vi "Read Body.vi"(8 "error in (no error)":errorcluster, 11 "Request in":refnum<class "Request.lvclass">) -> (0 "error out":errorcluster, 3 "Request out":refnum<class "Request.lvclass">)   [LabVIEW 2023, in "Request.lvclass"]
uses:
  Request.lvclass
  Request.lvclass/Request.ctl
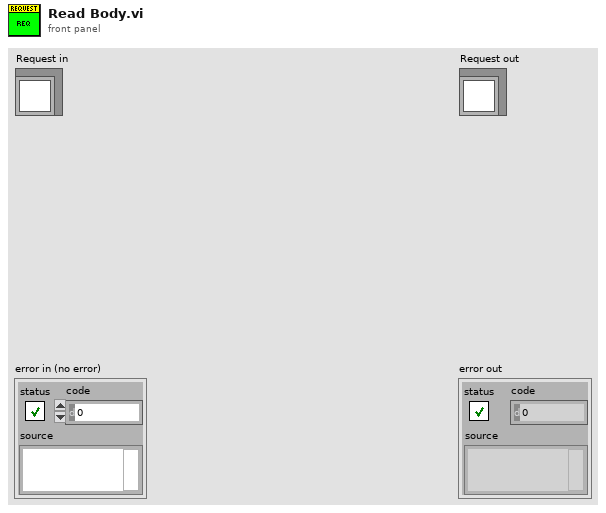
[diagram p1: front panel]
types:
  T1 = enum16{"Standard", "Buffered", "CRLF", "Immediate"}
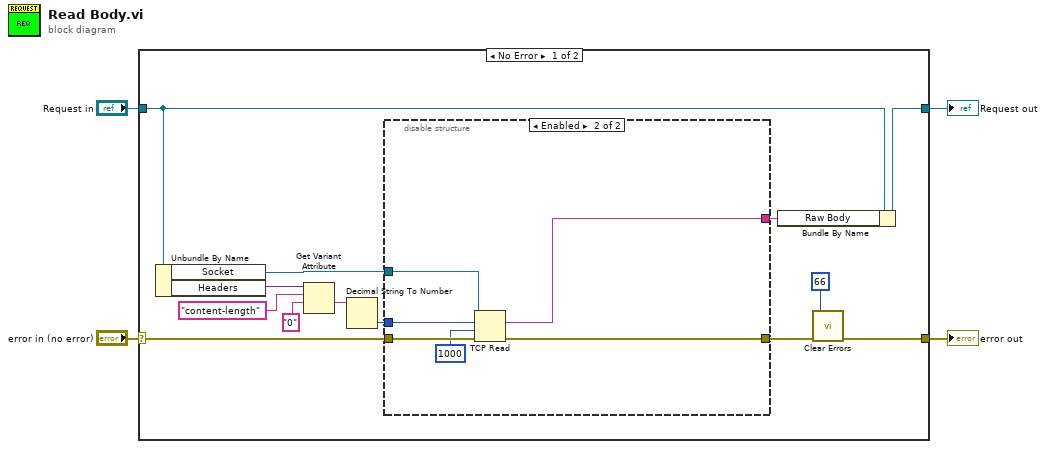
[diagram p0: block diagram]
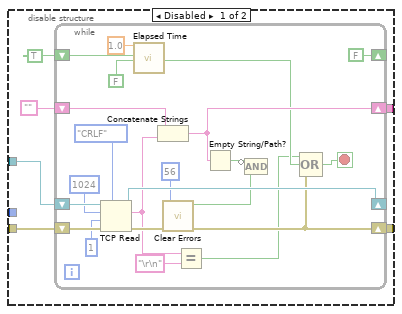
[diagram p2: hidden frame]
diagram:
  n1 = case shown="No Error" "error in (no error)" {
    selector: "error in (no error)" -> [w17 w53]
    tunnel: [w11 w53] -> w3
    tunnel: [w14 w52] -> w1
    tunnel: "Request in" -> [w15 w52]
    frame No Error {
      n2 = Unbundle By Name(w15) -> ("Socket"=w10:refnum<k5>, "Headers"=w9:variant)
      n3 = Get Variant Attribute(Variant=w9, name="content-length" ("y"), default value (empty Variant)="0" ("y")) -> (value=w6:string)  [unwired: 1 in, 3 out]
      n4 = Decimal String To Number(string=w6) -> (number=w5:i32)  [unwired: 2 in, 1 out]
      n5 = disable-structure shown="Enabled" {
        disable-tunnel: w17 -> [w23 w51]
        disable-tunnel: [w21 w48] -> w16
        disable-tunnel: [w20 w47] -> w12
        disable-tunnel: w10 -> [w18 w50]
        disable-tunnel: w5 -> [_ w49]
        frame Disabled {
          n6 = while {
            shift-right: [w34] -> w21
            shift-left: "" -> [w41]
            shift-right: [w39] -> _
            shift-left: w18 -> [w45]
            shift-right: [w35] -> w20
            shift-left: w23 -> [w44]
            shift-right: [FALSE ("Auto Reset")] -> _
            shift-left: TRUE ("Auto Reset") -> [w30]
            stop <- w37 stop-if-true
            n7 = TCP Read(connection ID=w45, bytes to read=1024, error in (no error)=w44, 7:T1."CRLF" ("mode (standard)"), 9:1 ("timeout ms (wait forever: -1)")) -> (connection ID out=w39:refnum<k5>, data out=w25:string, error out=w38:errorcluster)
            n8 = call "Elapsed Time"("Time Target (s)"=1.0, "Reset"=w30, "Auto Reset"=FALSE) -> ("Time has Elapsed"=w29:bool)  [unwired: 9 in, 7 out]
            n9 = Concatenate Strings(w41, w25) -> (w34:string)
            n10 = call <vilib>:"Clear Errors.vi"("error in (no error)"=w38, "specific error code to clear (0: all)"=56 ("bytes to read")) -> ("error out"=w35:errorcluster, "specific error cleared?"=w32:bool)  [unwired: 4 in]
            n11 = Equal?(x=w25, y="\r\n") -> (x = y?=w24:bool)
            n12 = Empty String/Path?(string/path=w34) -> (empty?=w33:bool)
            n13 = Compound Arithmetic op=AND(invert w33, w32) -> ()  [unwired: 1 out]
            n14 = Compound Arithmetic op=OR(w24, w29, w35) -> (w37:bool)
          }
        }
        frame Enabled {
          n15 = TCP Read(connection ID=w50, bytes to read=w49, error in (no error)=w51, 9:1000 ("timeout ms (25000)")) -> (data out=w48:string, error out=w47:errorcluster)  [unwired: 1 in, 1 out]
        }
      }
      n16 = Bundle By Name(cluster=w15, "Raw Body"=w16) -> (w14:refnum<class "Request.lvclass">)
      n17 = call <vilib>:"Clear Errors.vi"("error in (no error)"=w12, "specific error code to clear (0: all)"=66 ("bytes to read")) -> ("error out"=w11:errorcluster)  [unwired: 4 in, 1 out]
    }
    frame Error {
    }
  }
  "error out" <- w3
  "Request out" <- w1
